vi "Create Node Config.vi"(8 "error in (no error)":errorcluster, 11 "Volatus Core in":refnum<class "Volatus Core.lvclass">) -> (0 "error out":errorcluster, 2 "Node":refnum<class "Node Config.lvclass">, 3 "Volatus Core out":refnum<class "Volatus Core.lvclass">)   [LabVIEW 2020, in "Volatus.lvlib" / "Volatus Core.lvclass"]
uses:
  Volatus Core.lvclass
  Volatus Core.lvclass/Volatus Core.ctl
  VolatusConfig/Node/Node.lvclass
  lv-vecto/Vecto/Node Config/Node Config.lvclass
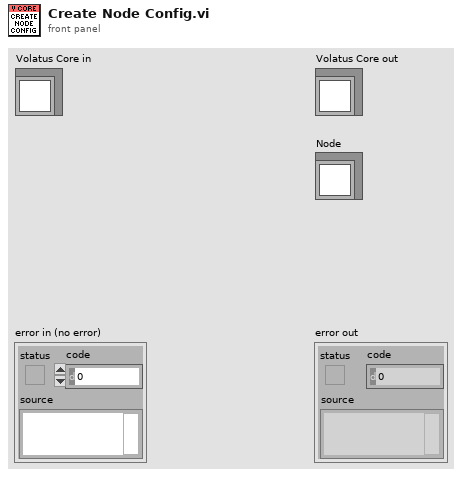
[diagram p1: front panel]
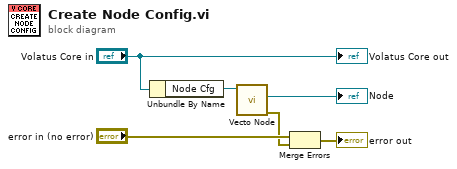
[diagram p0: block diagram]
diagram:
  n1 = Unbundle By Name("Volatus Core in") -> ("Node Cfg"=w5:refnum<class "Node.lvclass">)
  n2 = call "Vecto Node.vi"("Node in"=w5) -> ("error out"=w1:errorcluster, "Vecto Node"=→"Node":refnum<class "Node Config.lvclass">)  [unwired: 8 in, 1 out]
  n3 = Merge Errors("error in (no error)", w1) -> (→"error out":errorcluster)
  "Volatus Core out" <- "Volatus Core in"
